vi "TestIOs.vi"() -> ()   [LabVIEW 2011]
panel:
  in  "stop":bool
  out "All Tags":cluster{"Tags":string[], "Values":dbl[]}
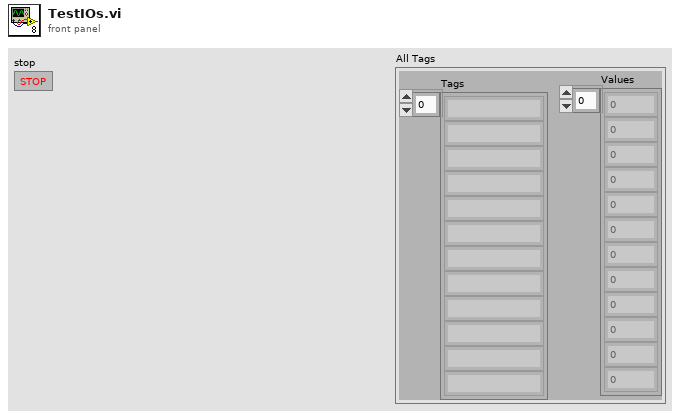
[diagram p1: front panel]
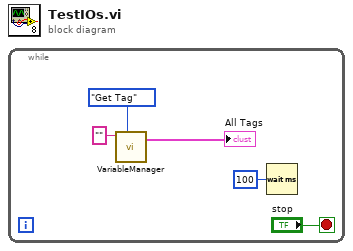
[diagram p0: block diagram]
diagram:
  n1 = while {
    stop <- "stop" stop-if-true
    n2 = call "VariableManager.vi"("Operation"=enum16{"Get Tag", "Set Tag"}."Get Tag", "Tag"="") -> ("All Tags"=→"All Tags":cluster{"Tags":string[], "Values":dbl[]})  [unwired: 1 in, 8 out]
    n3 = Wait (ms)(milliseconds to wait=u32 100) -> ()  [unwired: 1 out]
  }
